vi "Replace Named Format Specifier.vi"(8 "error in (no error)":errorcluster, 10 "data":variant, 11 "format string":string) -> (0 "error out":errorcluster, 3 "resulting string":string)   [LabVIEW 2018, in "Logging.lvlib" / "Format String.lvclass"]
uses:
  Format String.lvclass
  <vilib>/regexp/Match Regular Expression.xnode
  <vilib>/ErrorRing/Error Ring.xnode
  <vilib>/Utility/Data Type/NI_Data Type.lvlib
panel:
  # "Connector Pane"
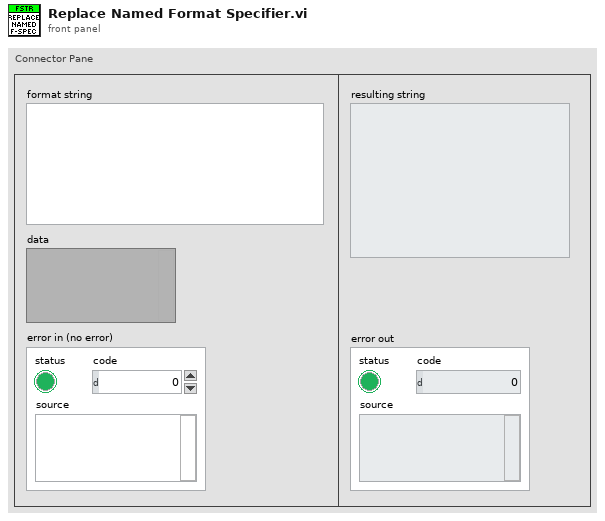
[diagram p1: front panel]
types:
  T1 = typedef "NI_Data Type.lvlib/Data Type.ctl" = enum8{"Invalid Type", "Void", "I8", "I16", "I32", "I64", "U8", "U16", "U32", "U64", "Single Float", "Double Float", "Extended Float", "Single Complex", "Double Complex", "Extended Complex", "Enum U8", "Enum U16", "Enum U32", "Enum U64", "Single Float With Unit", "Double Float With Unit", "Extended Float With Unit", "Single Complex with Unit", "Double Complex with Unit", "Extended Complex with Unit", "Boolean", "String", "Path", "Picture", "Tag", "Array", "Cluster", "Variant", "LV Variant", "Waveform", "Timestamp", "Digital Waveform", "Digital Data", "ExpressData", "Refnum", "External Data", "VI", "Poly VI", "LabVIEW Class Instance", "Fixed Point", "Set Collection", "Map Collection"}
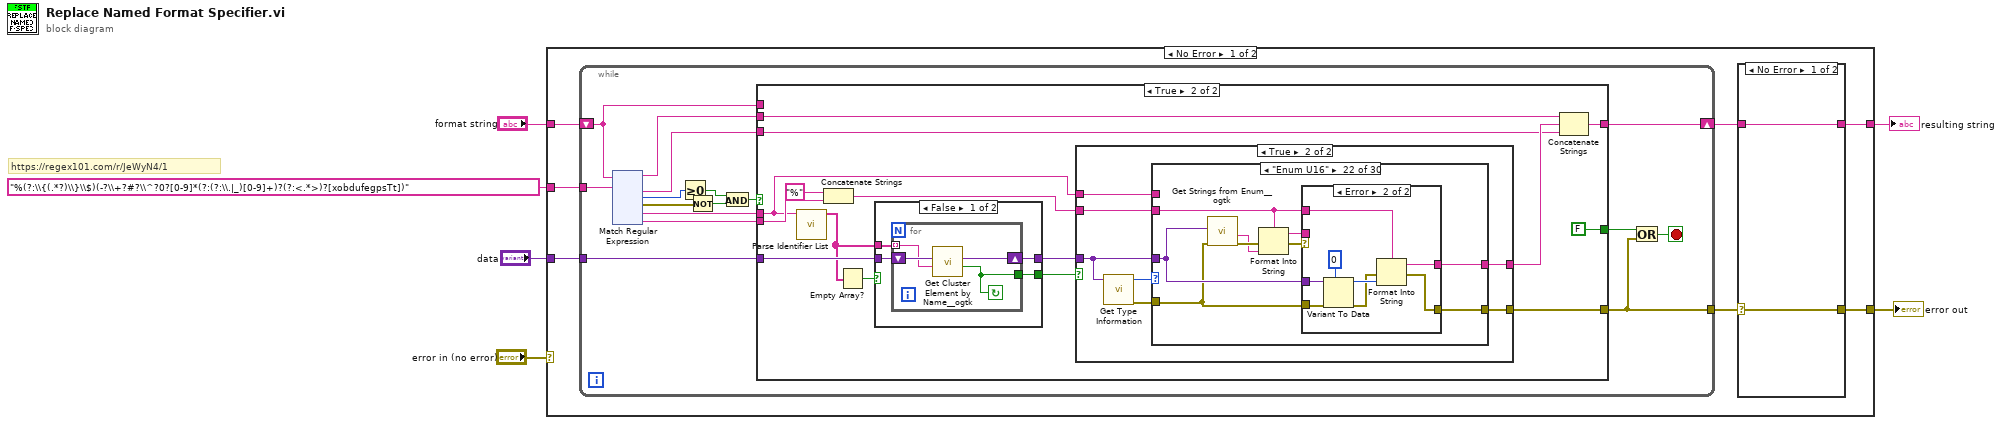
[diagram p0: block diagram]
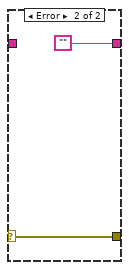
[diagram p2: hidden frame]
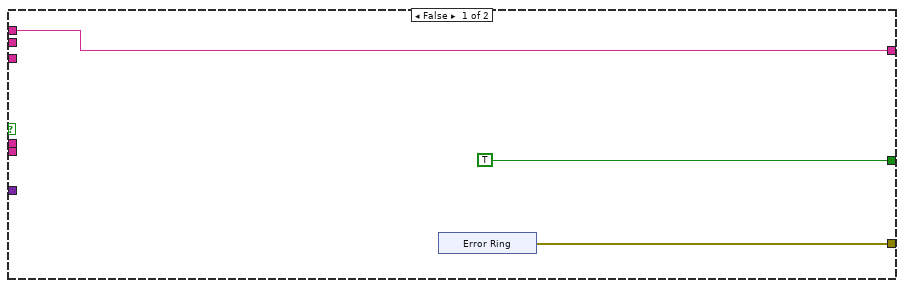
[diagram p3: hidden frame]
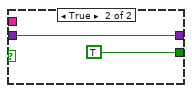
[diagram p4: hidden frame]
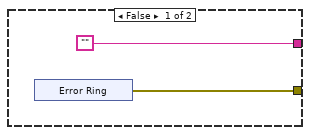
[diagram p5: hidden frame]
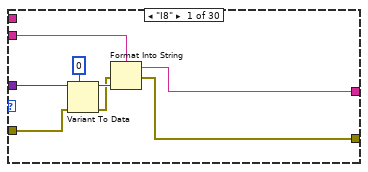
[diagram p6: hidden frame]
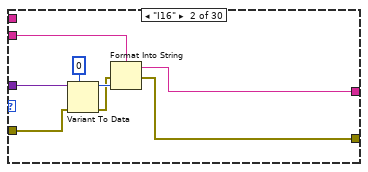
[diagram p7: hidden frame]
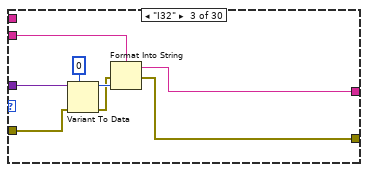
[diagram p8: hidden frame]
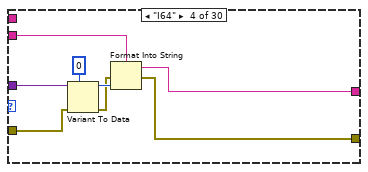
[diagram p9: hidden frame]
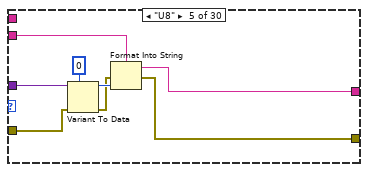
[diagram p10: hidden frame]
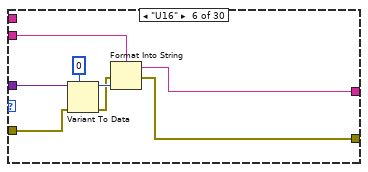
[diagram p11: hidden frame]
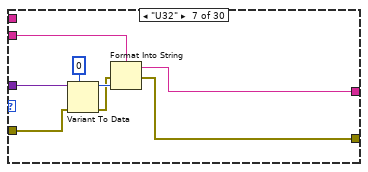
[diagram p12: hidden frame]
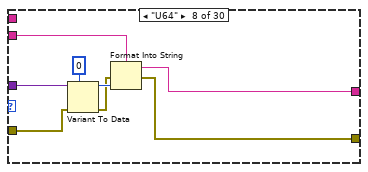
[diagram p13: hidden frame]
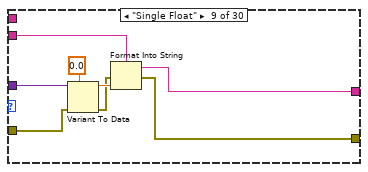
[diagram p14: hidden frame]
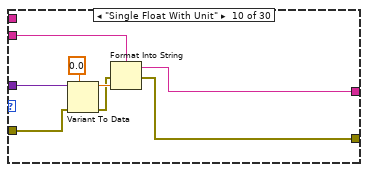
[diagram p15: hidden frame]
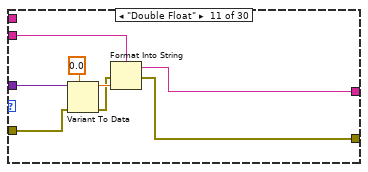
[diagram p16: hidden frame]
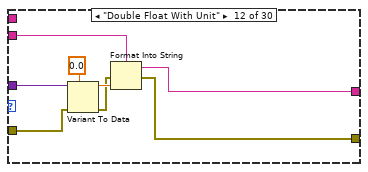
[diagram p17: hidden frame]
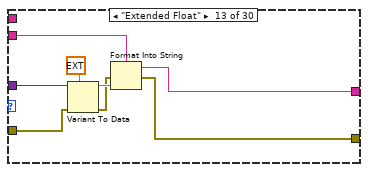
[diagram p18: hidden frame]
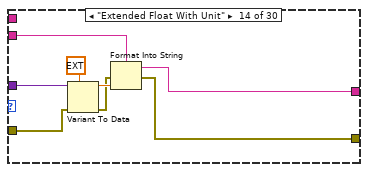
[diagram p19: hidden frame]
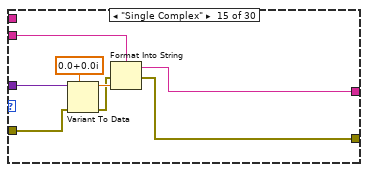
[diagram p20: hidden frame]
diagram:
  # "https://regex101.com/r/JeWyN4/1"
  n1 = case shown="No Error" "error in (no error)" {
    selector: "error in (no error)" -> [_ w465]
    tunnel: "format string" -> [w13 _]
    tunnel: "%(?:\\{(.*?)\\}\\$)(-?\\+?#?\\^?0?[0-9]*(?:(?:\\.|_)[0-9]+)?(?:<.*>)?[xobdufegpsTt])" -> [w12 _]
    tunnel: "data" -> [w11 _]
    tunnel: [w9 w465] -> w3
    tunnel: [w8 ""] -> w2
    frame No Error {
      n2 = while {
        tunnel: w12 -> [w32]
        tunnel: w11 -> [w30]
        shift-right: [w27] -> w7
        shift-left: w13 -> [w18]
        tunnel: [w19] -> w10
        stop <- w20 stop-if-true
        n3 = xnode "Match Regular Expression"("input string"=w18, "regular expression"=w32) -> ("before match"=w29:string, "after match"=w28:string, "offset past match"=w26:i32, "error out"=w25:errorcluster, "submatch 1"=w33:string, "submatch 2"=w31:string)  [unwired: 4 in, 1 out]
        n4 = Greater Or Equal To 0?(x=w26) -> (x >= 0?=w24:bool)
        n5 = Not(x=w25) -> (.not. x?=w23:bool)
        n6 = And(x=w24, y=w23) -> (x .and. y?=w22:bool)
        n7 = case shown="True" w22 {
          tunnel: w33 -> [_ w160]
          tunnel: w31 -> [_ w171]
          tunnel: w30 -> [_ w161]
          tunnel: w29 -> [_ w167]
          tunnel: w28 -> [_ w165]
          tunnel: [w156 w164] -> w27
          tunnel: [TRUE FALSE] -> w21
          tunnel: [w154 w162] -> w19
          tunnel: w18 -> [w156 _]
          frame False {
            n8 = xnode "Error Ring"() -> ("error out"=w154:errorcluster)
          }
          frame True {
            n9 = call "Parse Identifier List.vi"("string"=w160) -> ("identifier list"=w159:string[])  [unwired: 10 in]
            n10 = Concatenate Strings("%" ("string"), w171) -> (w168:string)
            n11 = Empty Array?(array=w159) -> (empty?=w158:bool)
            n12 = case shown="False" w158 {
              tunnel: w159 -> [w176 _]
              tunnel: [w175 TRUE ("found?")] -> w170
              tunnel: [w174 w182] -> w169
              tunnel: w161 -> [w173 w182]
              frame False {
                n13 = for {
                  tunnel: w176 -> [w179] mode=indexing
                  shift-right: [w178] -> w174
                  shift-left: w173 -> [w180]
                  tunnel: [w177] -> w175
                  stop <- w177 continue-if-true
                  n14 = call <userlib>:"Get Cluster Element by Name__ogtk.vi"("Element Name"=w179, "Cluster"=w180) -> ("found?"=w177:bool, "VElement"=w178:variant)  [unwired: 7 in, 1 out]
                }
              }
              frame True {
              }
            }
            n15 = case shown="True" w170 {
              tunnel: w169 -> [_ w190]
              tunnel: ["" w191] -> w166
              tunnel: w168 -> [_ w189]
              tunnel: [w183 w188] -> w162
              tunnel: w160 -> [_ w187]
              frame False {
                n16 = xnode "Error Ring"() -> ("error out"=w183:errorcluster)
              }
              frame True {
                n17 = call <vilib>:"Get Type Information.vi"("variant"=w190) -> ("error out"=w186:errorcluster, "type"=w192:T1)  [unwired: 6 in, 3 out]
                n18 = case shown="\"Enum U16\"" w192 {
                  tunnel: [w195 w203 w211 w219 w227 w235 w243 w251 w259 w267 w275 w283 w291 w299 w307 w315 w323 w331 w339 w347 w356 w375 w394 w413 w431 w439 w447 w455 "" ""] -> w191
                  tunnel: w190 -> [w200 w208 w216 w224 w232 w240 w248 w256 w264 w272 w280 w288 w296 w304 w312 w320 w328 w336 w344 w352 w359 w378 w397 w416 w436 w444 w452 w460 _ _]
                  tunnel: w189 -> [w198 w206 w214 w222 w230 w238 w246 w254 w262 w270 w278 w286 w294 w302 w310 w318 w326 w334 w342 w350 w358 w377 w396 w415 w434 w442 w450 w458 _ _]
                  tunnel: [w196 w204 w212 w220 w228 w236 w244 w252 w260 w268 w276 w284 w292 w300 w308 w316 w324 w332 w340 w348 w354 w373 w392 w411 w432 w440 w448 w456 w461 w463] -> w188
                  tunnel: w187 -> [_ _ _ _ _ _ _ _ _ _ _ _ _ _ _ _ _ _ _ _ _ _ _ _ _ _ _ _ _ _]
                  tunnel: w186 -> [w193 w201 w209 w217 w225 w233 w241 w249 w257 w265 w273 w281 w289 w297 w305 w313 w321 w329 w337 w345 w353 w372 w391 w410 w429 w437 w445 w453 w461 w463]
                  frame "I8" {
                    n19 = Variant To Data(error in=w193, type=i8 0, Variant=w200) -> (data=w197:i8, error out=w194:errorcluster)
                    n20 = Format Into String(format string=w198, error in=w194, w197) -> (resulting string=w195:string, error out=w196:errorcluster)  [unwired: 1 in]
                  }
                  frame "I16" {
                    n21 = Variant To Data(error in=w201, type=i16 0, Variant=w208) -> (data=w205:i16, error out=w202:errorcluster)
                    n22 = Format Into String(format string=w206, error in=w202, w205) -> (resulting string=w203:string, error out=w204:errorcluster)  [unwired: 1 in]
                  }
                  frame "I32" {
                    n23 = Variant To Data(error in=w209, type=0, Variant=w216) -> (data=w213:i32, error out=w210:errorcluster)
                    n24 = Format Into String(format string=w214, error in=w210, w213) -> (resulting string=w211:string, error out=w212:errorcluster)  [unwired: 1 in]
                  }
                  frame "I64" {
                    n25 = Variant To Data(error in=w217, type=i64 0, Variant=w224) -> (data=w221:i64, error out=w218:errorcluster)
                    n26 = Format Into String(format string=w222, error in=w218, w221) -> (resulting string=w219:string, error out=w220:errorcluster)  [unwired: 1 in]
                  }
                  frame "U8" {
                    n27 = Variant To Data(error in=w225, type=u8 0, Variant=w232) -> (data=w229:u8, error out=w226:errorcluster)
                    n28 = Format Into String(format string=w230, error in=w226, w229) -> (resulting string=w227:string, error out=w228:errorcluster)  [unwired: 1 in]
                  }
                  frame "U16" {
                    n29 = Variant To Data(error in=w233, type=u16 0, Variant=w240) -> (data=w237:u16, error out=w234:errorcluster)
                    n30 = Format Into String(format string=w238, error in=w234, w237) -> (resulting string=w235:string, error out=w236:errorcluster)  [unwired: 1 in]
                  }
                  frame "U32" {
                    n31 = Variant To Data(error in=w241, type=u32 0, Variant=w248) -> (data=w245:u32, error out=w242:errorcluster)
                    n32 = Format Into String(format string=w246, error in=w242, w245) -> (resulting string=w243:string, error out=w244:errorcluster)  [unwired: 1 in]
                  }
                  frame "U64" {
                    n33 = Variant To Data(error in=w249, type=u64 0, Variant=w256) -> (data=w253:u64, error out=w250:errorcluster)
                    n34 = Format Into String(format string=w254, error in=w250, w253) -> (resulting string=w251:string, error out=w252:errorcluster)  [unwired: 1 in]
                  }
                  frame "Single Float" {
                    n35 = Variant To Data(error in=w257, type=sgl 0.0, Variant=w264) -> (data=w261:sgl, error out=w258:errorcluster)
                    n36 = Format Into String(format string=w262, error in=w258, w261) -> (resulting string=w259:string, error out=w260:errorcluster)  [unwired: 1 in]
                  }
                  frame "Single Float With Unit" {
                    n37 = Variant To Data(error in=w265, type=sgl 0.0, Variant=w272) -> (data=w269:sgl, error out=w266:errorcluster)
                    n38 = Format Into String(format string=w270, error in=w266, w269) -> (resulting string=w267:string, error out=w268:errorcluster)  [unwired: 1 in]
                  }
                  frame "Double Float" {
                    n39 = Variant To Data(error in=w273, type=0.0, Variant=w280) -> (data=w277:dbl, error out=w274:errorcluster)
                    n40 = Format Into String(format string=w278, error in=w274, w277) -> (resulting string=w275:string, error out=w276:errorcluster)  [unwired: 1 in]
                  }
                  frame "Double Float With Unit" {
                    n41 = Variant To Data(error in=w281, type=0.0, Variant=w288) -> (data=w285:dbl, error out=w282:errorcluster)
                    n42 = Format Into String(format string=w286, error in=w282, w285) -> (resulting string=w283:string, error out=w284:errorcluster)  [unwired: 1 in]
                  }
                  frame "Extended Float" {
                    n43 = Variant To Data(error in=w289, type=ext 0.0, Variant=w296) -> (data=w293:ext, error out=w290:errorcluster)
                    n44 = Format Into String(format string=w294, error in=w290, w293) -> (resulting string=w291:string, error out=w292:errorcluster)  [unwired: 1 in]
                  }
                  frame "Extended Float With Unit" {
                    n45 = Variant To Data(error in=w297, type=ext 0.0, Variant=w304) -> (data=w301:ext, error out=w298:errorcluster)
                    n46 = Format Into String(format string=w302, error in=w298, w301) -> (resulting string=w299:string, error out=w300:errorcluster)  [unwired: 1 in]
                  }
                  frame "Single Complex" {
                    n47 = Variant To Data(error in=w305, type=csg 0.0+0.0i, Variant=w312) -> (data=w309:csg, error out=w306:errorcluster)
                    n48 = Format Into String(format string=w310, error in=w306, w309) -> (resulting string=w307:string, error out=w308:errorcluster)  [unwired: 1 in]
                  }
                  frame "Single Complex with Unit" {
                    n49 = Variant To Data(error in=w313, type=csg 0.0+0.0i, Variant=w320) -> (data=w317:csg, error out=w314:errorcluster)
                    n50 = Format Into String(format string=w318, error in=w314, w317) -> (resulting string=w315:string, error out=w316:errorcluster)  [unwired: 1 in]
                  }
                  frame "Double Complex" {
                    n51 = Variant To Data(error in=w321, type=cdb 0.0+0.0i, Variant=w328) -> (data=w325:cdb, error out=w322:errorcluster)
                    n52 = Format Into String(format string=w326, error in=w322, w325) -> (resulting string=w323:string, error out=w324:errorcluster)  [unwired: 1 in]
                  }
                  frame "Double Complex with Unit" {
                    n53 = Variant To Data(error in=w329, type=cdb 0.0+0.0i, Variant=w336) -> (data=w333:cdb, error out=w330:errorcluster)
                    n54 = Format Into String(format string=w334, error in=w330, w333) -> (resulting string=w331:string, error out=w332:errorcluster)  [unwired: 1 in]
                  }
                  frame "Extended Complex" {
                    n55 = Variant To Data(error in=w337, type=cxt 0.0+0.0i, Variant=w344) -> (data=w341:cxt, error out=w338:errorcluster)
                    n56 = Format Into String(format string=w342, error in=w338, w341) -> (resulting string=w339:string, error out=w340:errorcluster)  [unwired: 1 in]
                  }
                  frame "Extended Complex with Unit" {
                    n57 = Variant To Data(error in=w345, type=cxt 0.0+0.0i, Variant=w352) -> (data=w349:cxt, error out=w346:errorcluster)
                    n58 = Format Into String(format string=w350, error in=w346, w349) -> (resulting string=w347:string, error out=w348:errorcluster)  [unwired: 1 in]
                  }
                  frame "Enum U8" {
                    n59 = call <userlib>:"Get Strings from Enum__ogtk.vi"("error in (no error)"=w353, "Enum"=w359) -> ("error out"=w361:errorcluster, "String Value"=w360:string)  [unwired: 6 in, 2 out]
                    n60 = Format Into String(format string=w358, error in=w361, w360) -> (resulting string=w355:string, error out=w357:errorcluster)  [unwired: 1 in]
                    n61 = case shown="Error" w357 {
                      selector: w357 -> [w362 _]
                      tunnel: w359 -> [_ w371]
                      tunnel: w358 -> [_ w367]
                      tunnel: [w363 w366] -> w356
                      tunnel: w355 -> [w363 _]
                      tunnel: [w362 w365] -> w354
                      tunnel: w353 -> [_ w364]
                      frame No Error {
                      }
                      frame Error {
                        n62 = Variant To Data(error in=w364, type=u8 0, Variant=w371) -> (data=w370:u8, error out=w368:errorcluster)
                        n63 = Format Into String(format string=w367, error in=w368, w370) -> (resulting string=w366:string, error out=w365:errorcluster)  [unwired: 1 in]
                      }
                    }
                  }
                  frame "Enum U16" {
                    n64 = call <userlib>:"Get Strings from Enum__ogtk.vi"("error in (no error)"=w372, "Enum"=w378) -> ("error out"=w380:errorcluster, "String Value"=w379:string)  [unwired: 6 in, 2 out]
                    n65 = Format Into String(format string=w377, error in=w380, w379) -> (resulting string=w374:string, error out=w376:errorcluster)  [unwired: 1 in]
                    n66 = case shown="Error" w376 {
                      selector: w376 -> [w381 _]
                      tunnel: w378 -> [_ w390]
                      tunnel: w377 -> [_ w386]
                      tunnel: [w382 w385] -> w375
                      tunnel: w374 -> [w382 _]
                      tunnel: [w381 w384] -> w373
                      tunnel: w372 -> [_ w383]
                      frame No Error {
                      }
                      frame Error {
                        n67 = Variant To Data(error in=w383, type=u16 0, Variant=w390) -> (data=w389:u16, error out=w387:errorcluster)
                        n68 = Format Into String(format string=w386, error in=w387, w389) -> (resulting string=w385:string, error out=w384:errorcluster)  [unwired: 1 in]
                      }
                    }
                  }
                  frame "Enum U32" {
                    n69 = call <userlib>:"Get Strings from Enum__ogtk.vi"("error in (no error)"=w391, "Enum"=w397) -> ("error out"=w399:errorcluster, "String Value"=w398:string)  [unwired: 6 in, 2 out]
                    n70 = Format Into String(format string=w396, error in=w399, w398) -> (resulting string=w393:string, error out=w395:errorcluster)  [unwired: 1 in]
                    n71 = case shown="Error" w395 {
                      selector: w395 -> [w400 _]
                      tunnel: w397 -> [_ w409]
                      tunnel: w396 -> [_ w405]
                      tunnel: [w401 w404] -> w394
                      tunnel: w393 -> [w401 _]
                      tunnel: [w400 w403] -> w392
                      tunnel: w391 -> [_ w402]
                      frame No Error {
                      }
                      frame Error {
                        n72 = Variant To Data(error in=w402, type=u32 0, Variant=w409) -> (data=w408:u32, error out=w406:errorcluster)
                        n73 = Format Into String(format string=w405, error in=w406, w408) -> (resulting string=w404:string, error out=w403:errorcluster)  [unwired: 1 in]
                      }
                    }
                  }
                  frame "Enum U64" {
                    n74 = call <userlib>:"Get Strings from Enum__ogtk.vi"("error in (no error)"=w410, "Enum"=w416) -> ("error out"=w418:errorcluster, "String Value"=w417:string)  [unwired: 6 in, 2 out]
                    n75 = Format Into String(format string=w415, error in=w418, w417) -> (resulting string=w412:string, error out=w414:errorcluster)  [unwired: 1 in]
                    n76 = case shown="Error" w414 {
                      selector: w414 -> [w419 _]
                      tunnel: w416 -> [_ w428]
                      tunnel: w415 -> [_ w424]
                      tunnel: [w420 w423] -> w413
                      tunnel: w412 -> [w420 _]
                      tunnel: [w419 w422] -> w411
                      tunnel: w410 -> [_ w421]
                      frame No Error {
                      }
                      frame Error {
                        n77 = Variant To Data(error in=w421, type=u64 0, Variant=w428) -> (data=w427:u64, error out=w425:errorcluster)
                        n78 = Format Into String(format string=w424, error in=w425, w427) -> (resulting string=w423:string, error out=w422:errorcluster)  [unwired: 1 in]
                      }
                    }
                  }
                  frame "Boolean" {
                    n79 = Variant To Data(error in=w429, type=FALSE, Variant=w436) -> (data=w433:bool, error out=w430:errorcluster)
                    n80 = Format Into String(format string=w434, error in=w430, w433) -> (resulting string=w431:string, error out=w432:errorcluster)  [unwired: 1 in]
                  }
                  frame "String" {
                    n81 = Variant To Data(error in=w437, type="", Variant=w444) -> (data=w441:string, error out=w438:errorcluster)
                    n82 = Format Into String(format string=w442, error in=w438, w441) -> (resulting string=w439:string, error out=w440:errorcluster)  [unwired: 1 in]
                  }
                  frame "Path" {
                    n83 = Variant To Data(error in=w445, type=path "", Variant=w452) -> (data=w449:path, error out=w446:errorcluster)
                    n84 = Format Into String(format string=w450, error in=w446, w449) -> (resulting string=w447:string, error out=w448:errorcluster)  [unwired: 1 in]
                  }
                  frame "Timestamp" {
                    n85 = Variant To Data(error in=w453, type=timestamp(0 s since 1904-01-01), Variant=w460) -> (data=w457:timestamp, error out=w454:errorcluster)
                    n86 = Format Into String(format string=w458, error in=w454, w457) -> (resulting string=w455:string, error out=w456:errorcluster)  [unwired: 1 in]
                  }
                  frame "Void" {
                  }
                  frame Default {
                  }
                }
              }
            }
            n87 = Concatenate Strings(w167, w166, w165) -> (w164:string)
          }
        }
        n88 = Or(x=w21, y=w19) -> (x .or. y?=w20:bool)
      }
      n89 = case shown="No Error" w10 {
        selector: w10 -> [w15 w17]
        tunnel: [w15 w17] -> w9
        tunnel: [w14 ""] -> w8
        tunnel: w7 -> [w14 _]
        frame No Error {
        }
        frame Error {
        }
      }
    }
    frame Error {
    }
  }
  "resulting string" <- w2
  "error out" <- w3
